vi "methane_reactor_update.vi"(10 "spec_file":path) -> (2 "spec_file_dup":path)   [LabVIEW 2019]
uses:
  lib/libSimulationControl/libSimulationControl.lvlib
  lib/libFileFunctions/libFileFunctions.lvlib
panel:
  out "outflow_file":path
  # "*******************************************************************\nBiogas Plant Control\n\nAuthor: Paul Zügel\nGCSC-Frankfurt am Main 2020\n\n*******************************************************************"
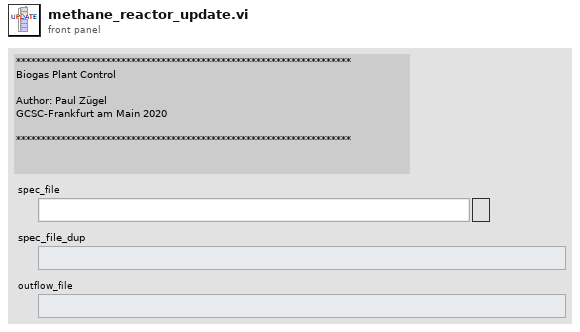
[diagram p1: front panel]
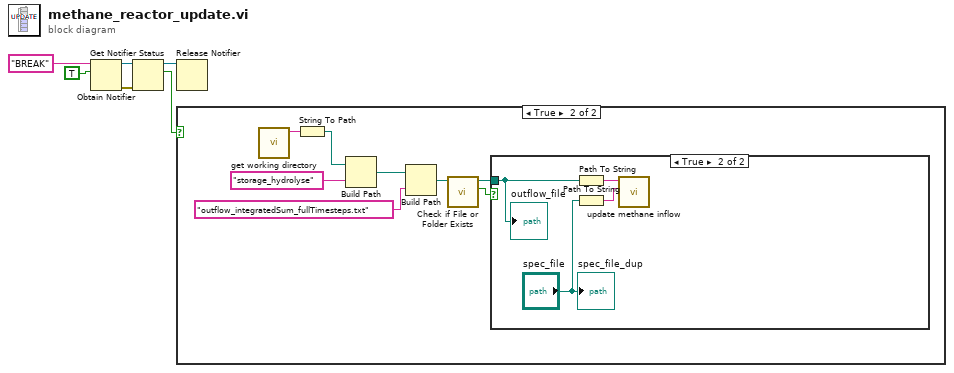
[diagram p0: block diagram]
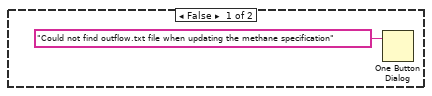
[diagram p3: hidden frame]
diagram:
  n1 = Obtain Notifier(name (unnamed)="BREAK", notification data type=TRUE) -> (notifier out=w4:refnum<notifier>, error out=w3:errorcluster)  [unwired: 2 in, 1 out]
  n2 = Get Notifier Status(notifier=w4, error in (no error)=w3) -> (notifier out=w1:refnum<notifier>, current notification=w2:bool)  [unwired: 3 out]
  n3 = Release Notifier(notifier=w1) -> ()  [unwired: 2 in, 3 out]
  n4 = case shown="True" w2 {
    frame False {
    }
    frame True {
      n5 = call "get working directory.vi"() -> ("function return"=w11:string)  [unwired: 10 in, 1 out]
      n6 = String To Path(string=w11) -> (path=w10:path)
      n7 = Build Path(base path=w10, name or relative path="storage_hydrolyse") -> (appended path=w13:path)
      n8 = Build Path(base path=w13, name or relative path="outflow_integratedSum_fullTimesteps.txt") -> (appended path=w9:path)
      n9 = call <vilib>:"Check if File or Folder Exists.vi"("path"=w9) -> ("file or folder exists?"=w7:bool, "dup path"=w8:path)  [unwired: 8 in, 1 out]
      n10 = case shown="True" w7 {
        tunnel: w8 -> [_ w19]
        frame False {
          n11 = One Button Dialog(message="Could not find outflow.txt file when updating the methane specification") -> ()  [unwired: 1 in, 1 out]
        }
        frame True {
          n12 = Path To String(path=w19) -> (string=w17:string)
          n13 = Path To String(path="spec_file") -> (string=w16:string)
          n14 = call "update methane inflow.vi"("methane_specfile"=w16, "outflow_infile"=w17) -> ()  [unwired: 9 in, 1 out]
          "spec_file_dup" <- "spec_file"
          "outflow_file" <- w19
        }
      }
    }
  }
